vi "Read MonochromatorRanges.vi"(8 "error in (no error)":errorcluster, 11 "MonoClientCommunicator in":refnum<class "MonoClientCommunicator.lvclass">) -> (0 "error out":errorcluster, 2 "MonochromatorRanges":T1, 3 "MonoClientCommunicator out":refnum<class "MonoClientCommunicator.lvclass">)   [LabVIEW 2016, in "MonoClientCommunicator.lvclass"]
uses:
  MonoClientCommunicator.lvclass
  ts_sallv_atmonochromator/VIs/MonochromatorRanges.ctl
  MonoClientCommunicator.lvclass/MonoClientCommunicator.ctl
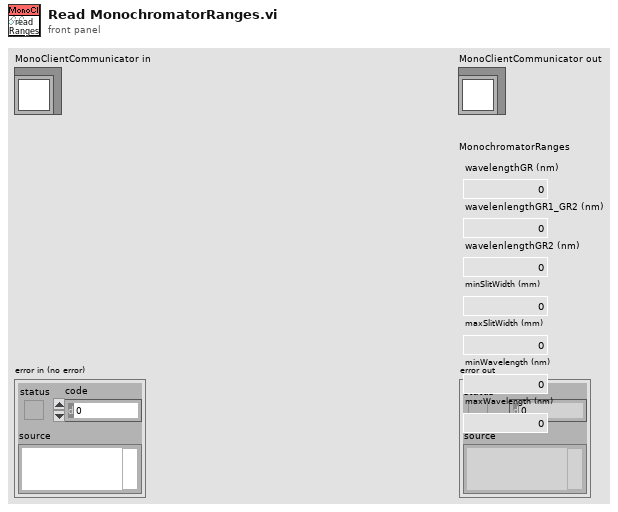
[diagram p1: front panel]
types:
  T1 = typedef "MonochromatorRanges.ctl" = cluster{"maxWavelength (nm)":sgl, "minWavelength (nm)":sgl, "maxSlitWidth (mm)":sgl, "minSlitWidth (mm)":sgl, "wavelenlengthGR2 (nm)":sgl, "wavelenlengthGR1_GR2 (nm)":sgl, "wavelengthGR (nm)":sgl}
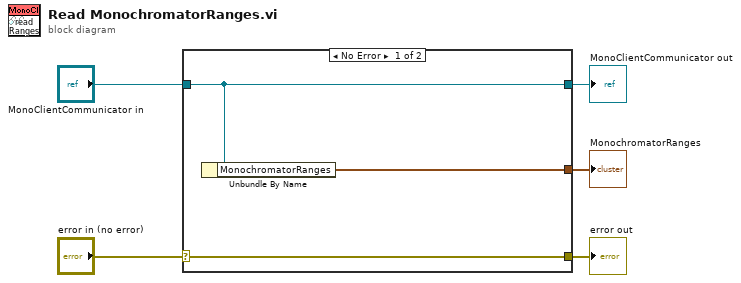
[diagram p0: block diagram]
diagram:
  n1 = case shown="No Error" "error in (no error)" {
    selector: "error in (no error)" -> [w8 w9]
    tunnel: [w8 w9] -> w4
    tunnel: [w7 w10] -> w2
    tunnel: "MonoClientCommunicator in" -> [w7 w10]
    tunnel: [w6 _] -> w1
    frame No Error {
      n2 = Unbundle By Name(w7) -> ("MonochromatorRanges"=w6:T1)
    }
    frame Error {
    }
  }
  "error out" <- w4
  "MonoClientCommunicator out" <- w2
  "MonochromatorRanges" <- w1
